vi "Frequency_IPDFT.vi"(8 "error in":errorcluster, 9 "Estimation Model":string(combo)="power", 10 "Fs":dbl, 11 "Signal":dbl[](array[numeric])) -> (0 "error out":errorcluster, 2 "A":dbl, 3 "f":dbl)   [LabVIEW 2014]
uses:
  <vilib>/imath/engines/lvmath/Plug In/_Char/NIMS_CH_character datatype.ctl
  <vilib>/imath/engines/lvmath/Plug In/_Char/NIMS_CH_String to Character Array.vi
  <vilib>/imath/engines/lvmath2/RunTimeEngine/BuiltInFunctions/size/NIMS_I32=size(GRow,I32).vi
  <instcachedir>/0/NIMS_I32=size(GRow,I32)_4662369BBD5B4B51BF0F6B31B2927178.lvgen/NIMS_I32=size(GRow,I32)_4662369BBD5B4B51BF0F6B31B2927178_000.vi
  <vilib>/imathl/engines/lvmath/Functions/Error Handling/Create Error.vi
  <vilib>/imath/engines/lvmath2/RunTimeEngine/RangeToken/NIMS_Range.vi
  <instcachedir>/0/NIMS_Range_9BCE657718DF4976A877346C61F22738.lvgen/NIMS_Range_9BCE657718DF4976A877346C61F22738_001.vi
  <vilib>/imath/engines/lvmath2/RunTimeEngine/ArithmeticOperatorToken/NIMS_ArithmeticOperator_times.vi
  <instcachedir>/0/NIMS_ArithmeticOperator_times_2EFF5B13FCA4492A81D59089AD809F54.lvgen/NIMS_ArithmeticOperator_times_2EFF5B13FCA4492A81D59089AD809F54_000.vi
  <vilib>/imath/engines/lvmath2/RunTimeEngine/BuiltInFunctions/fft/NIMS_fft(GV).vi
  <instcachedir>/0/NIMS_fft(GV)_4C6467FC22F84E4BA42517A07EF978B0.lvgen/NIMS_fft(GV)_4C6467FC22F84E4BA42517A07EF978B0_000.vi
  <vilib>/imath/engines/lvmath2/RunTimeEngine/ErrorHandling/NIMS_Error From Error Code.vi
  <instcachedir>/0/NIMS_Range_9BCE657718DF4976A877346C61F22738.lvgen/NIMS_Range_9BCE657718DF4976A877346C61F22738_000.vi
  <vilib>/imath/engines/lvmath2/RunTimeSupport/NIMS_Error if Not Equal.vi
  <instcachedir>/0/NIMS_Error if Not Equal_8A0E9F659B9142D69417CC259581C4FD.lvgen/NIMS_Error if Not Equal_8A0E9F659B9142D69417CC259581C4FD_001.vi
  <vilib>/imath/engines/lvmath2/RunTimeEngine/IndexRead/NIMS V(V).vi
  <instcachedir>/0/NIMS V(V)_298D9CB7BFEB42B8BC8D9C3C28AE8C70.lvgen/NIMS V(V)_298D9CB7BFEB42B8BC8D9C3C28AE8C70_001.vi
  <vilib>/imath/engines/lvmath2/RunTimeEngine/BuiltInFunctions/max/1 input/NIMS_max(CV).vi
  <instcachedir>/0/NIMS_max(CV)_C6F6073AFB634DD3BED44AE26C6E4AAB.lvgen/NIMS_max(CV)_C6F6073AFB634DD3BED44AE26C6E4AAB_000.vi
  <vilib>/imath/engines/lvmath2/RunTimeEngine/ErrorHandling/NIMS_Create Error From Enums.vi
  <vilib>/imath/engines/lvmath2/RunTimeEngine/IndexRead/NIMS V(S).vi
  <instcachedir>/0/NIMS V(S)_0488751826AF41519A22953C041130DC.lvgen/NIMS V(S)_0488751826AF41519A22953C041130DC_003.vi
  <vilib>/imath/engines/lvmath2/RunTimeEngine/BuiltInFunctions/abs/NIMS_abs(signed).vi
  <instcachedir>/0/NIMS_abs(signed)_C4FCB8E6058B49B797C7C8D53CA5F6EC.lvgen/NIMS_abs(signed)_C4FCB8E6058B49B797C7C8D53CA5F6EC_002.vi
  <vilib>/imath/engines/lvmath/Plug In/_Char/NIMS_CH_Character 2D to String 1D.vi
  <vilib>/imath/engines/lvmath2/RunTimeEngine/BuiltInFunctions/strcmp/NIMS_strcmp.vi
  <vilib>/imath/engines/lvmath2/RunTimeEngine/ArithmeticOperatorToken/NIMS_ArithmeticOperator_power(S).vi
  <instcachedir>/0/NIMS_ArithmeticOperator_power(S)_CAFE680B12A64A3A8F5E28A20C679B7D.lvgen/NIMS_ArithmeticOperator_power(S)_CAFE680B12A64A3A8F5E28A20C679B7D_014.vi
  <instcachedir>/0/NIMS_ArithmeticOperator_power(S)_CAFE680B12A64A3A8F5E28A20C679B7D.lvgen/NIMS_ArithmeticOperator_power(S)_CAFE680B12A64A3A8F5E28A20C679B7D_010.vi
  <instcachedir>/0/NIMS_ArithmeticOperator_power(S)_CAFE680B12A64A3A8F5E28A20C679B7D.lvgen/NIMS_ArithmeticOperator_power(S)_CAFE680B12A64A3A8F5E28A20C679B7D_009.vi
  <vilib>/imath/engines/lvmath2/RunTimeEngine/VariableToken/NIMS_VariableToken_CondDefined.vi
  <instcachedir>/0/NIMS_VariableToken_CondDefined_EE8DD211A89249938CE6537267F5C9B3.lvgen/NIMS_VariableToken_CondDefined_EE8DD211A89249938CE6537267F5C9B3_006.vi
  <vilib>/imath/engines/lvmath2/RunTimeEngine/BuiltInFunctions/angle/NIMS_angle.vi
  <instcachedir>/0/NIMS_angle_6DDAE2BD99E0421EB990B6436E94D88F.lvgen/NIMS_angle_6DDAE2BD99E0421EB990B6436E94D88F_003.vi
  <vilib>/imath/engines/lvmath2/RunTimeEngine/NodeEndStatement/NIMS_NodeEndStatement_Output.vi
  <instcachedir>/0/NIMS_NodeEndStatement_Output_53EC0D466D134D7ABD903AC30B43404B.lvgen/NIMS_NodeEndStatement_Output_53EC0D466D134D7ABD903AC30B43404B_010.vi
  <instcachedir>/0/NIMS_NodeEndStatement_Output_53EC0D466D134D7ABD903AC30B43404B.lvgen/NIMS_NodeEndStatement_Output_53EC0D466D134D7ABD903AC30B43404B_001.vi
  <vilib>/imath/engines/lvmath2/RunTimeEngine/ErrorHandling/NIMS_Finalize Error.vi
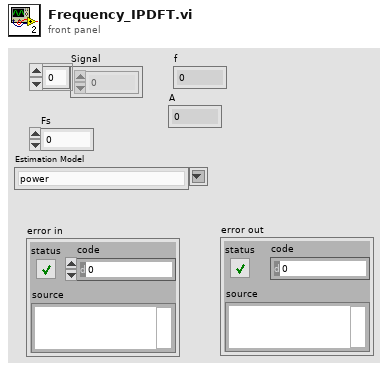
[diagram p1: front panel]
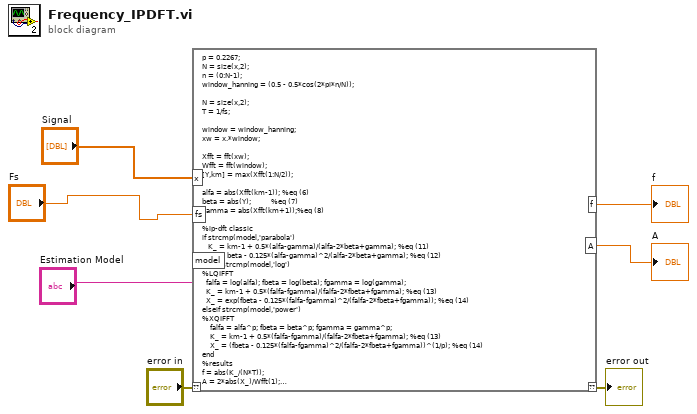
[diagram p0: block diagram]
diagram:
  n1 = mathscript code="p = 0.2267;\nN = size(x,2);\nn = (0:N-1);\nwindow_hanning = (0.5 - 0.5*cos(2*pi*n/N));\n\nN = size(x,2);\nT = 1/fs;\n\nwindow = window_hanning;\nxw = x.*window;\n\nXfft = fft(xw);\nWfft = fft(window);\n[Y,km] = max(Xfft(1:N/2));\n\nalfa = abs(Xfft(km-1)); %eq (6)\nbeta = abs(Y);          %eq (7)\ngamma = abs(Xfft(km+1));%eq (8)\n\n%ip-dft classic\nif strcmp(model,'parabola')\n   K_ = km-1 + 0.5*(alfa-gamma)/(alfa-2*beta+gamma); %eq (11)\n   X_ = beta - 0.125*(alfa-gamma)^2/(alfa-2*beta+gamma); %eq (12)\nelseif strcmp(model,'log')\n%LQIFFT\n  falfa = log(alfa); fbeta = log(beta); fgamma = log(gamma);\n  K_ = km-1 + 0.5*(falfa-fgamma)/(falfa-2*fbeta+fgamma); %eq (13)\n  X_ = exp(fbeta - 0.125*(falfa-fgamma)^2/(falfa-2*fbeta+fgamma)); %eq (14)\nelseif strcmp(model,'power')\n%XQIFFT\n    falfa = alfa^p; fbeta = beta^p; fgamma = gamma^p;\n    K_ = km-1 + 0.5*(falfa-fgamma)/(falfa-2*fbeta+fgamma); %eq (13)\n    X_ = (fbeta - 0.125*(falfa-fgamma)^2/(falfa-2*fbeta+fgamma))^(1/p); %eq (14)\nend\n%results\nf = abs(K_/(N*T));\nA = 2*abs(X_)/Wfft(1);\nph = angle(Xfft(km-1));"("??"="error in", "x"="Signal", "fs"="Fs", "model"="Estimation Model") -> ("??"=→"error out":errorcluster, "f"=→"f":dbl, "A"=→"A":cdb)
